vi "TargetVolFillTime.vi"(6 "Target Gallons":dbl, 7 "Temperature Valve Control":T1(ring), 8 "Error In":errorcluster, 9 "GEA Inputs":T2 {"Destination" format="%.0x"; "Source" format="%.0x"}, 10 "Standalone?":bool, 11 "GEA2 Reference In":refnum<k24>) -> (0 "Error Out":errorcluster, 1 "Target Gallon Fill Time (sec)":dbl, 3 "GEA2 Reference Out":refnum<k24>)   [LabVIEW 2016, in "TLMB.lvlib"]
uses:
  Projects/TLMB.lvlib
  Q:/Common/DLLs/GEA3/GeaCommunication.dll
  Common/DLLs/GEA3/GeaCommunication.dll
  Common/LabVIEW GEA2 Toolkit/LabVIEW_GEA2_Toolkit.lvlibp/type defs/Source_Destination.ctl
  Common/LabVIEW GEA2 Toolkit/LabVIEW_GEA2_Toolkit.lvlibp/type defs/ERD Read Data In.ctl
  Common/LabVIEW GEA2 Toolkit/LabVIEW_GEA2_Toolkit.lvlibp/type defs/Data Type.ctl
  Common/LabVIEW GEA2 Toolkit/LabVIEW_GEA2_Toolkit.lvlibp/type defs/ERD Write Data In.ctl
  type defs/Fixed Valve Control.ctl
  type defs/User Selected Temperature.ctl
  Common/LabVIEW GEA2 Toolkit/LabVIEW_GEA2_Toolkit.lvlibp
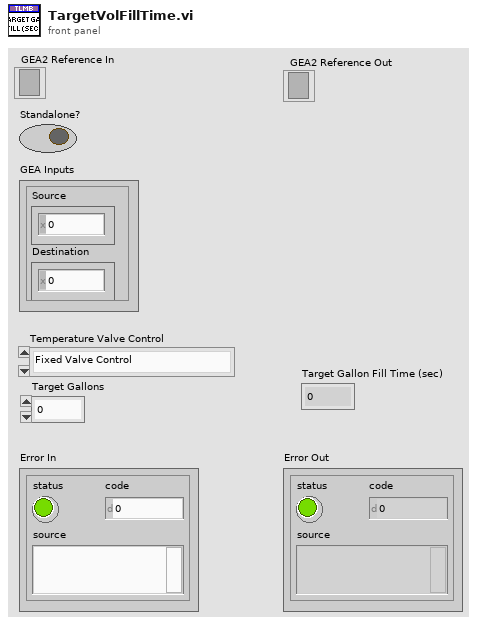
[diagram p1: front panel]
types:
  T1 = enum16{"Fixed Valve Control", "Temperature Option Valve Control"}
  T2 = typedef "LabVIEW_GEA2_Toolkit.lvlibp/Source_Destination.ctl" = cluster{"Source":u8, "Destination":u8}
  T3 = typedef "LabVIEW_GEA2_Toolkit.lvlibp/ERD Read Data In.ctl" = cluster{"ERD Number":u16, "Data Type":T4}
  T4 = typedef "LabVIEW_GEA2_Toolkit.lvlibp/Data Type.ctl" = enum16{"string", "boolean", "uint8_t", "uint16_t", "uint32_t", "uint64_t", "int8_t", "int16_t", "int32_t", "int64_t"}
  T5 = typedef "LabVIEW_GEA2_Toolkit.lvlibp/ERD Write Data In.ctl" = cluster{"ERD Number":u16, "Data Type":T4, "Data":string}
  T6 = typedef "TLMB.lvlib/Fixed Valve Control.ctl" = enum16{"Warm Valve", "Hot Valve", "Cold Valve"}
  T7 = typedef "TLMB.lvlib/User Selected Temperature.ctl" = enum16{"Tap Cold", "Cold", "Cool", "Colors", "Warm", "Hot"}
  T8 = typedef "LabVIEW_GEA2_Toolkit.lvlibp/ERD Read Data Out.ctl" = cluster{"ERD Number":u16, "Data":string}
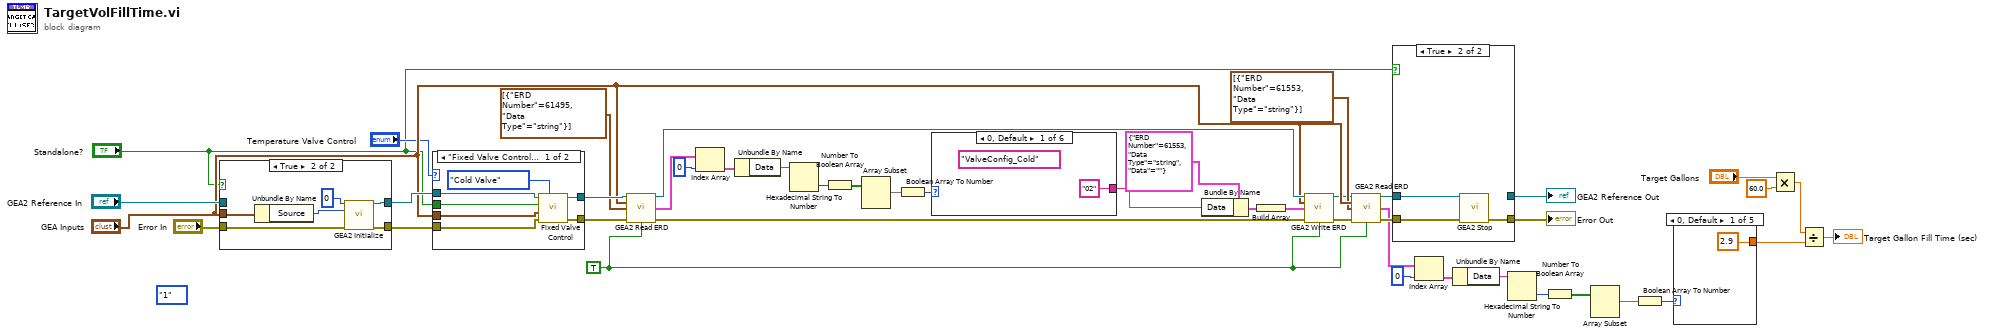
[diagram p0: block diagram]
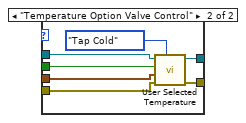
[diagram p2: hidden frame]
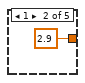
[diagram p3: hidden frame]
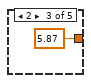
[diagram p4: hidden frame]
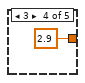
[diagram p5: hidden frame]
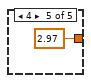
[diagram p6: hidden frame]
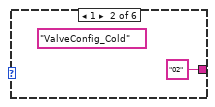
[diagram p7: hidden frame]
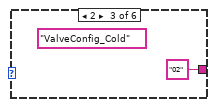
[diagram p8: hidden frame]
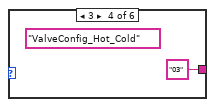
[diagram p9: hidden frame]
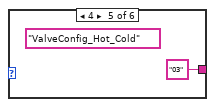
[diagram p10: hidden frame]
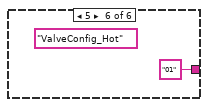
[diagram p11: hidden frame]
diagram:
  (unwired) enum32{"8", "4", "3", "2", "1"}."1"
  w20 = TRUE ("Verify ERD Response?")
  n1 = case shown="True" "Standalone?" {
    tunnel: "Error In" -> [w46 w53]
    tunnel: [w46 w52] -> w45
    tunnel: "GEA2 Reference In" -> [w47 _]
    tunnel: [w47 w51] -> w40
    tunnel: "GEA Inputs" -> [_ w49]
    frame False {
    }
    frame True {
      n2 = Unbundle By Name(w49) -> ("Source"=w50:u8)
      n3 = call "GEA2 Initialize.vi"("Board Index"=0, "Source Address"=w50, "error in"=w53) -> ("GEA2 Reference Out"=w51:refnum<k24>, "error out"=w52:errorcluster)  [unwired: 10 in, 1 out]
    }
  }
  n4 = case shown="\"Fixed Valve Control\", Default" "Temperature Valve Control" {
    tunnel: w45 -> [w57 w67]
    tunnel: w40 -> [w59 w66]
    tunnel: [w58 w65] -> w39
    tunnel: [w56 w64] -> w38
    tunnel: "GEA Inputs" -> [w55 w63]
    tunnel: "Standalone?" -> [w54 w61]
    frame "Fixed Valve Control", Default {
      n5 = call "Fixed Valve Control.vi"("Fixed  Valve Control"=Fixed_Valve_Control."Cold Valve", "Error In"=w57, "GEA Inputs"=w55, "Standalone?"=w54, "GEA2 Reference In"=w59) -> ("Error Out"=w56:errorcluster, "GEA2 Reference Out"=w58:refnum<k24>)  [unwired: 5 in]
    }
    frame "Temperature Option Valve Control" {
      n6 = call "User Selected Temperature.vi"("User Selected Temperature"=User_Selected_Temperature."Tap Cold", "Error In"=w67, "GEA Inputs"=w63, "Standalone?"=w61, "GEA2 Reference In"=w66) -> ("Error Out"=w64:errorcluster, "GEA2 Reference Out"=w65:refnum<k24>)  [unwired: 5 in]
    }
  }
  n7 = call "GEA2 Read ERD.vi"("GEA2 Reference In"=w39, "GEA Inputs"="GEA Inputs", "Read ERD List"=T3[] [{"ERD Number"=61495, "Data Type"=enum."string"}], "Error In"=w38, "Verify ERD Response?"=w20) -> ("GEA2 Reference Out"=w32:refnum<k24>, "ERD Data Out"=w36:T8[], "Error Out"=w31:errorcluster)  [unwired: 7 in, 1 out]
  n8 = Index Array(array=w36, index=0) -> (element=w34:T8)
  n9 = Unbundle By Name(w34) -> ("Data"=w33:string)
  n10 = Hexadecimal String To Number(string=w33) -> (number=w3:u32)  [unwired: 2 in, 1 out]
  n11 = Number To Boolean Array(number=w3) -> (Boolean array=w7:bool[])
  n12 = Array Subset(array=w7) -> (w8:bool[])  [unwired: 2 in]
  n13 = Boolean Array To Number(Boolean array=w8) -> (number=w6:u32)
  n14 = case shown="0, Default" w6 {
    tunnel: ["02" "02" "02" "03" "03" "01"] -> w29
    frame 0, Default {
      (unwired) "ValveConfig_Cold"
    }
    frame 1 {
      (unwired) "ValveConfig_Cold"
    }
    frame 2 {
      (unwired) "ValveConfig_Cold"
    }
    frame 3 {
      (unwired) "ValveConfig_Hot_Cold"
    }
    frame 4 {
      (unwired) "ValveConfig_Hot_Cold"
    }
    frame 5 {
      (unwired) "ValveConfig_Hot"
    }
  }
  n15 = Bundle By Name(cluster=T5 {"ERD Number"=61553, "Data Type"=enum."string", "Data"=""} ("ERD Write Data In"), "Data"=w29) -> (w28:T5)
  n16 = Build Array(w28) -> (w27:T5[])
  n17 = call "GEA2 Write ERD.vi"("GEA2 Reference In"=w32, "GEA Inputs"="GEA Inputs", "Write ERD List"=w27, "Error In"=w31, "Verify ERD Response?"=w20) -> ("GEA2 Reference Out"=w24:refnum<k24>, "Error Out"=w23:errorcluster)  [unwired: 8 in, 1 out]
  n18 = call "GEA2 Read ERD.vi"("GEA2 Reference In"=w24, "GEA Inputs"="GEA Inputs", "Read ERD List"=T3[] [{"ERD Number"=61553, "Data Type"=enum."string"}], "Error In"=w23, "Verify ERD Response?"=w20) -> ("GEA2 Reference Out"=w22:refnum<k24>, "ERD Data Out"=w12:T8[], "Error Out"=w21:errorcluster)  [unwired: 7 in, 1 out]
  n19 = case shown="True" "Standalone?" {
    tunnel: w21 -> [w74 w78]
    tunnel: [w74 w77] -> w43
    tunnel: w22 -> [w75 w76]
    tunnel: [w75 _] -> w41
    frame False {
    }
    frame True {
      n20 = call "GEA2 Stop.vi"("GEA2 Reference In"=w76, "Error In"=w78) -> ("Error Out"=w77:errorcluster)  [unwired: 13 in]
    }
  }
  "Error Out" <- w43
  "GEA2 Reference Out" <- w41
  n21 = Index Array(array=w12, index=0) -> (element=w18:T8)
  n22 = Unbundle By Name(w18) -> ("Data"=w15:string)
  n23 = Hexadecimal String To Number(string=w15) -> (number=w2:u32)  [unwired: 2 in, 1 out]
  n24 = Number To Boolean Array(number=w2) -> (Boolean array=w4:bool[])
  n25 = Array Subset(array=w4) -> (w5:bool[])  [unwired: 2 in]
  n26 = Boolean Array To Number(Boolean array=w5) -> (number=w1:u32)
  n27 = case shown="0, Default" w1 {
    tunnel: [2.9 2.9 5.87 2.9 2.97] -> w14
    frame 0, Default {
    }
    frame 1 {
    }
    frame 2 {
    }
    frame 3 {
    }
    frame 4 {
    }
  }
  n28 = Multiply(x="Target Gallons", y=60.0) -> (x*y=w16:dbl)
  n29 = Divide(x=w16, y=w14) -> (x/y=→"Target Gallon Fill Time (sec)":dbl)
